vi "GEvt-BackgroundThread.vi"() -> ()   [LabVIEW 2020, in "Communicable State Machine.lvlib"]
uses:
  Communicable State Machine.lvlib
  GEvt-RequestDef.ctl
  _CSM_GlobalLog_MSG.ctl
  _CSM_Response Source Message.ctl
  _CSM_GlobalLog_MSG_TYPE.ctl
panel:
  out "Count":i32
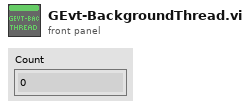
[diagram p1: front panel]
types:
  T1 = typedef "Communicable State Machine.lvlib/GEvt-RequestDef.ctl" = cluster{"Operation":enum16{"Obtain", "Destroy", "Force Destroy"}, "RespQ":refnum<queue>, "CSM Global Log Event":refnum<user-event>}
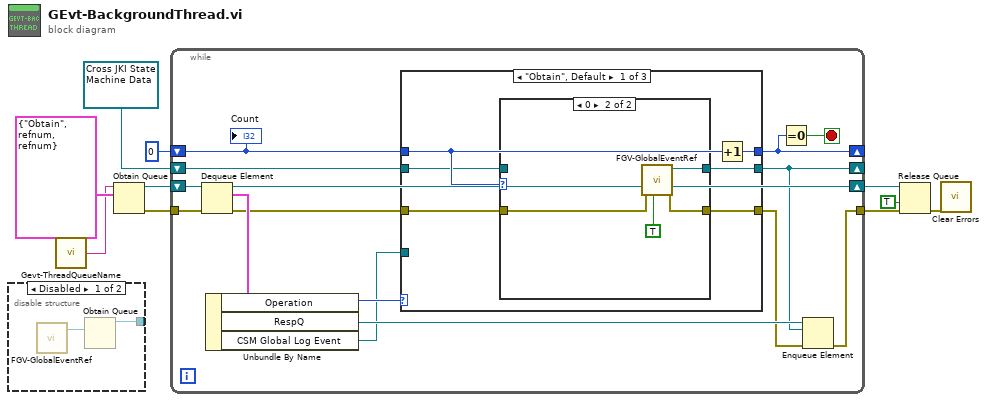
[diagram p0: block diagram]
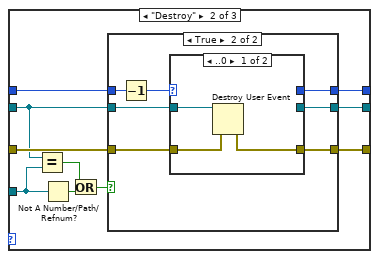
[diagram p4: hidden frame]
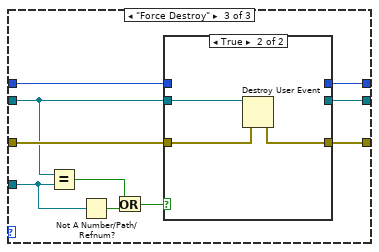
[diagram p7: hidden frame]
diagram:
  n1 = disable-structure shown="Disabled" {
    disable-tunnel: [w11 _] -> _
    frame Disabled {
      n2 = call "FGV-GlobalEventRef.vi"() -> ("CSM Global Log Event"=w12:refnum<user-event>)  [unwired: 10 in, 1 out]
      n3 = Obtain Queue(element data type=w12) -> (queue out=w11:refnum<queue>)  [unwired: 4 in, 2 out]
    }
    frame Enabled {
    }
  }
  n4 = call "Gevt-ThreadQueueName.vi"() -> ("ThreadQueueName"=w1:string)  [unwired: 5 in]
  n5 = Obtain Queue(name (unnamed)=w1, element data type=T1 {"Operation"=enum."Obtain", "RespQ"=refnum, "CSM Global Log Event"=refnum}) -> (queue out=w10:refnum<queue>, error out=w8:errorcluster)  [unwired: 3 in, 1 out]
  n6 = while {
    tunnel: w8 -> [w26]
    shift-right: [w23] -> w7
    shift-left: w10 -> [w27]
    tunnel: [w17] -> w6
    shift-right: [w15] -> _
    shift-left: 0 -> [w22]
    shift-right: [w14] -> _
    shift-left: refnum<user-event> refnum ("CSM Global Log Event") -> [w21]
    stop <- w16 stop-if-true
    n7 = Dequeue Element(queue=w27, error in (no error)=w26) -> (queue out=w23:refnum<queue>, element=w25:T1, error out=w19:errorcluster)  [unwired: 1 in, 1 out]
    n8 = Unbundle By Name(w25) -> ("Operation"=w24:enum16{"Obtain", "Destroy", "Force Destroy"}, "RespQ"=w20:refnum<queue>, "CSM Global Log Event"=w13:refnum<user-event>)
    n9 = case shown="\"Obtain\", Default" w24 {
      tunnel: [w33 w48 w72] -> w15
      tunnel: w22 -> [w32 w49 w71]
      tunnel: [w30 w47 w70] -> w14
      tunnel: w21 -> [w31 w41 w73]
      tunnel: w19 -> [w29 w46 w75]
      tunnel: [w28 w45 w74] -> w18
      tunnel: w13 -> [_ w42 w67]
      frame "Obtain", Default {
        n10 = case shown="0" w32 {
          tunnel: [w35 w39] -> w30
          tunnel: w31 -> [w35 _]
          tunnel: w29 -> [w34 w38]
          tunnel: [w34 w37] -> w28
          frame Default {
          }
          frame 0 {
            n11 = call "FGV-GlobalEventRef.vi"("Create(F)"=TRUE, "error in (no error)"=w38) -> ("error out"=w37:errorcluster, "CSM Global Log Event"=w39:refnum<user-event>)  [unwired: 8 in]
          }
        }
        n12 = Increment(x=w32) -> (x+1=w33:i32)
      }
      frame "Destroy" {
        n13 = Equal?(x=w41, y=w42) -> (x = y?=w44:bool)
        n14 = Not A Number/Path/Refnum?(number/path/refnum=w42) -> (NaN/Path/Refnum?=w43:bool)
        n15 = Or(x=w44, y=w43) -> (x .or. y?=w40:bool)
        n16 = case shown="True" w40 {
          tunnel: w49 -> [w52 w59]
          tunnel: [w52 w58] -> w48
          tunnel: [w51 w56] -> w47
          tunnel: w46 -> [w50 w55]
          tunnel: [w50 w54] -> w45
          tunnel: w41 -> [w51 w53]
          frame False {
          }
          frame True {
            n17 = Decrement(x=w59) -> (x-1=w57:i32)
            n18 = case shown="..0" w57 {
              selector: w57 -> [_ w65]
              tunnel: [_ w65] -> w58
              tunnel: [_ w64] -> w56
              tunnel: w53 -> [w62 w64]
              tunnel: w55 -> [w61 w63]
              tunnel: [w60 w63] -> w54
              frame ..0 {
                n19 = Destroy User Event(user event=w62, error in=w61) -> (error out=w60:errorcluster)
              }
              frame Default {
              }
            }
          }
        }
      }
      frame "Force Destroy" {
        n20 = Equal?(x=w73, y=w67) -> (x = y?=w69:bool)
        n21 = Not A Number/Path/Refnum?(number/path/refnum=w67) -> (NaN/Path/Refnum?=w68:bool)
        n22 = Or(x=w69, y=w68) -> (x .or. y?=w66:bool)
        n23 = case shown="True" w66 {
          tunnel: w75 -> [w78 w81]
          tunnel: [w78 w80] -> w74
          tunnel: w73 -> [w76 w79]
          tunnel: [w77 _] -> w72
          tunnel: w71 -> [w77 _]
          tunnel: [w76 _] -> w70
          frame False {
          }
          frame True {
            n24 = Destroy User Event(user event=w79, error in=w81) -> (error out=w80:errorcluster)
          }
        }
      }
    }
    n25 = Equal To 0?(x=w15) -> (x = 0?=w16:bool)
    n26 = Enqueue Element(queue=w20, element=w14, error in (no error)=w18) -> (error out=w17:errorcluster)  [unwired: 1 in, 2 out]
    "Count" <- w22
  }
  n27 = Release Queue(queue=w7, force destroy? (F)=TRUE, error in (no error)=w6) -> (error out=w2:errorcluster)  [unwired: 2 out]
  n28 = call "Clear Errors.vi"("error in (no error)"=w2) -> ()  [unwired: 5 in, 2 out]
